vi "Current File Paths.vi"(5 "Analysis Mode":T1, 6 "Local Data in":T3, 7 "UI Refs":T2, 8 "error in (no error)":errorcluster) -> (0 "error out":errorcluster, 2 "Distances":dbl[](array[numeric]), 3 "Tags":string[](array[string]))   [LabVIEW 2024]
uses:
  Controls/RVHR - Local Data.ctl
  Controls/Test Cluster.ctl
  Controls/Excluded Information.ctl
  Controls/Language.ctl
  Controls/Device_Type.ctl
  <vilib>/Utility/miscctls.llb/LVRectTypeDef.ctl
  <vilib>/Utility/miscctls.llb/LVBoundsTypeDef.ctl
  Controls/RVHR - UI Refs.ctl
  Controls/RVHR - Analysis Mode.ctl
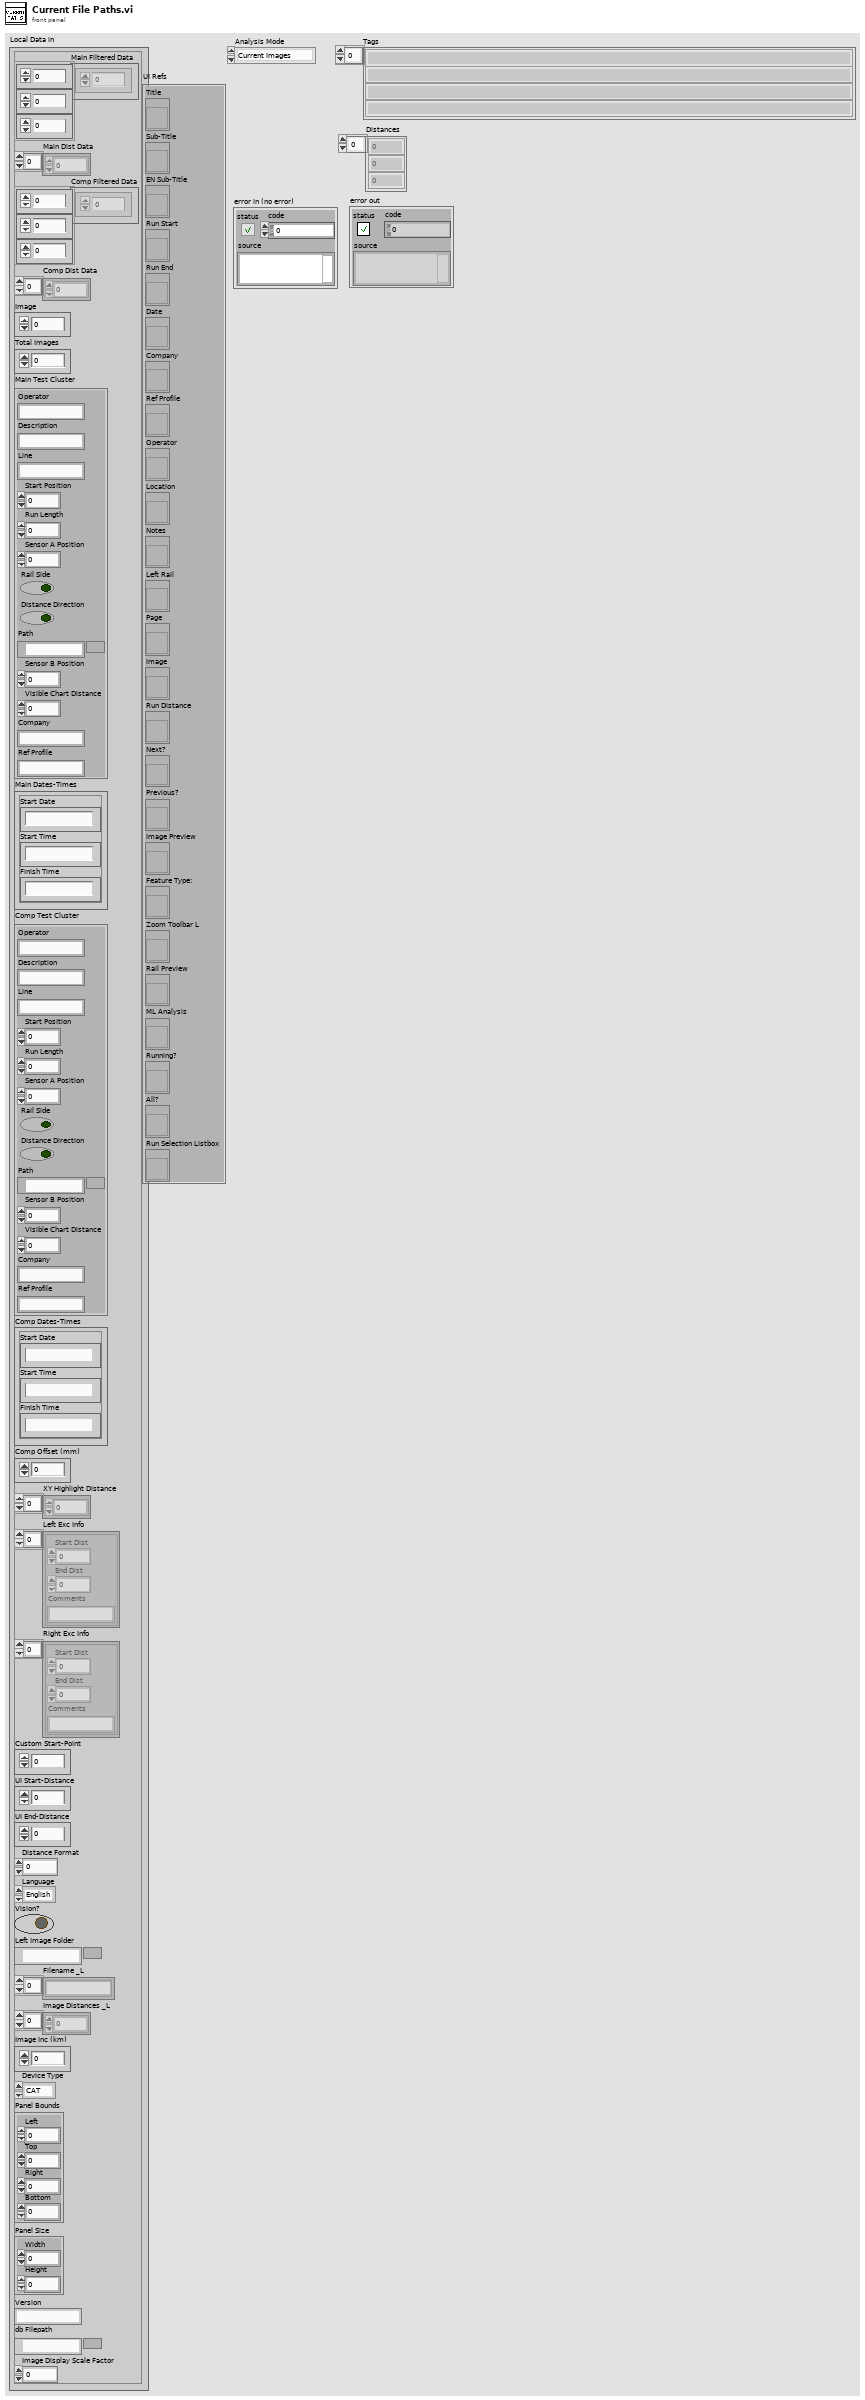
[diagram p1: front panel]
types:
  T1 = typedef "RVHR - Analysis Mode.ctl" = enum16{"Current Images", "Full Run"}
  T2 = typedef "RVHR - UI Refs.ctl" = cluster{"Title":refnum<vi>, "Sub-Title":refnum<vi>, "EN Sub-Title":refnum<vi>, "Run Start":refnum<vi>, "Run End":refnum<vi>, "Date":refnum<vi>, "Company":refnum<vi>, "Ref Profile":refnum<vi>, "Operator":refnum<vi>, "Location":refnum<vi>, "Notes":refnum<vi>, "Left Rail":refnum<vi>, "Page":refnum<vi>, "Image":refnum<vi>, "Run Distance":refnum<vi>, "Next?":refnum<vi>, "Previous?":refnum<vi>, "Image Preview":refnum<vi>, "Feature Type:":refnum<vi>, "Zoom Toolbar L":refnum<vi>, "Rail Preview":refnum<vi>, "ML Analysis":refnum<vi>, "Running?":refnum<vi>, "All?":refnum<vi>, "Run Selection Listbox":refnum<vi>}
  T3 = typedef "RVHR - Local Data.ctl" = cluster{"Main Filtered Data":dbl[][][], "Main Dist Data":dbl[], "Comp Filtered Data":dbl[][][], "Comp Dist Data":dbl[], "Image":u16, "Total Images":u16, "Main Test Cluster":T4, "Main Dates-Times":cluster{"Start Date":string, "Start Time":string, "Finish Time":string}, "Comp Test Cluster":T4, "Comp Dates-Times":cluster{"Start Date":string, "Start Time":string, "Finish Time":string}, "Comp Offset (mm)":i64, "XY Highlight Distance":dbl[], "Left Exc Info":T5[], "Right Exc Info":T5[], "Custom Start-Point":dbl, "UI Start-Distance":dbl, "UI End-Distance":dbl, "Distance Format":u8, "Language":T6, "Vision?":bool, "Left Image Folder":path, "Filename _L":string[], "Image Distances _L":dbl[], "Image Inc (km)":dbl, "Device Type":T7, "Panel Bounds":T8, "Panel Size":T9, "Version":string, "db Filepath":path, "Image Display Scale Factor":dbl}
  T4 = typedef "Test Cluster.ctl" = cluster{"Operator":string, "Description":string, "Line":string, "Start Position":dbl, "Run Length":dbl, "Sensor A Position":dbl, "Rail Side":bool, "Distance Direction":bool, "Path":path, "Sensor B Position":dbl, "Visible Chart Distance":dbl, "Company":string, "Ref Profile":string}
  T5 = typedef "Excluded Information.ctl" = cluster{"Start Dist":dbl, "End Dist":dbl, "Comments":string}
  T6 = typedef "Language.ctl" = enum16{"English", "Chinese", "German"}
  T7 = typedef "Device_Type.ctl" = enum16{"CAT", "Bi-CAT", "YRCA", "RCA", "RV-HR", "TV-HR"}
  T8 = typedef "LVRectTypeDef.ctl" = cluster{"Left":i16, "Top":i16, "Right":i16, "Bottom":i16}
  T9 = typedef "LVBoundsTypeDef.ctl" = cluster{"Width":u32, "Height":u32}
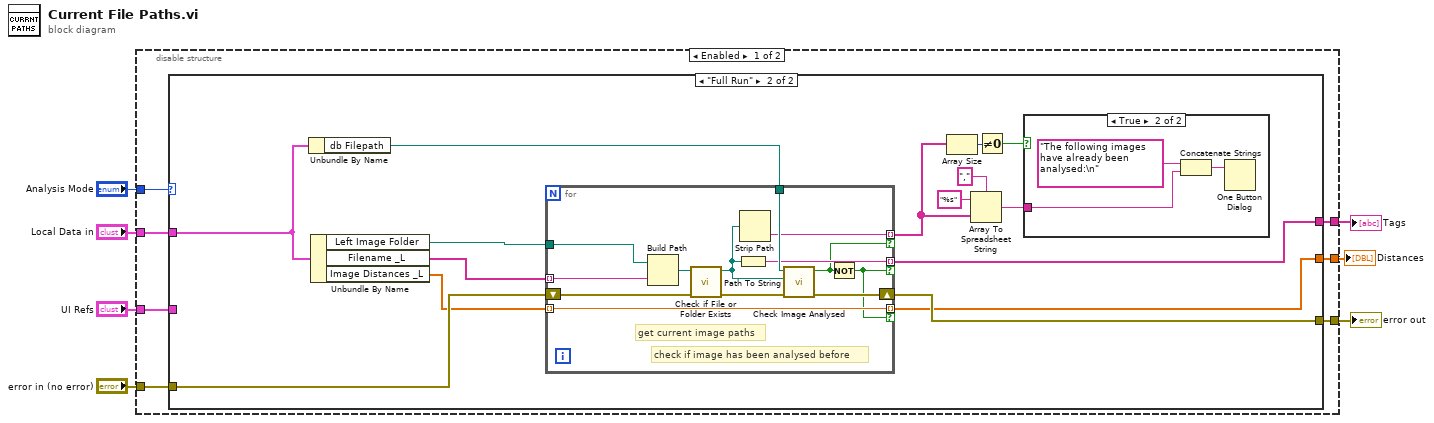
[diagram p0: block diagram]
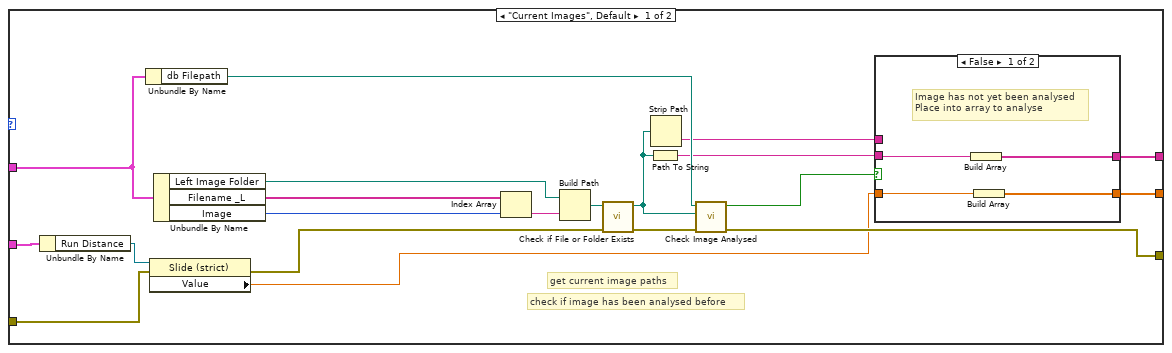
[diagram p2: hidden frame]
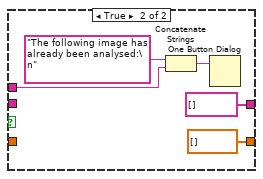
[diagram p3: hidden frame]
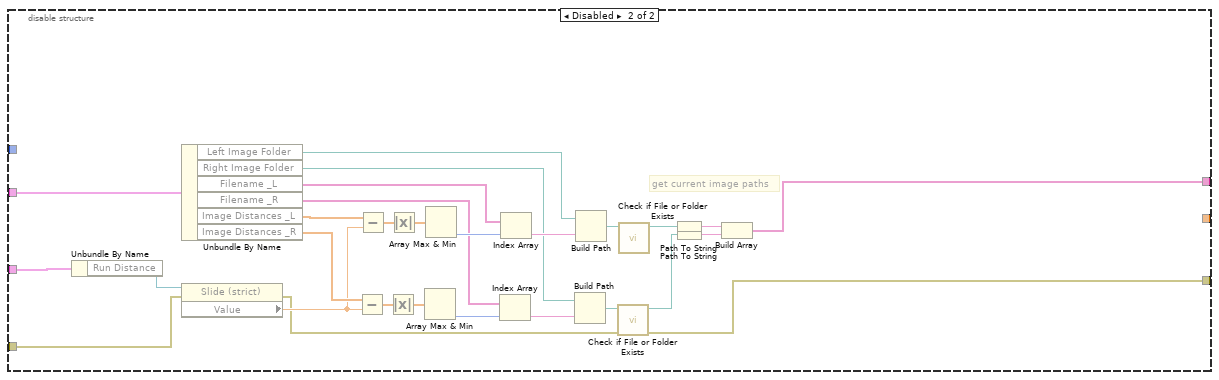
[diagram p5: hidden frame]
diagram:
  n1 = disable-structure shown="Enabled" {
    disable-tunnel: "Local Data in" -> [w10 w100]
    disable-tunnel: "UI Refs" -> [w14 w93]
    disable-tunnel: [w11 w78] -> w5
    disable-tunnel: [w12 w76] -> w4
    disable-tunnel: "error in (no error)" -> [w13 w75]
    disable-tunnel: "Analysis Mode" -> [w9 _]
    disable-tunnel: [w8 _] -> w1
    frame Enabled {
      n2 = case shown="\"Full Run\"" w9 {
        tunnel: w14 -> [w34 _]
        tunnel: w13 -> [w32 w58]
        tunnel: [w27 w55] -> w12
        tunnel: [w17 w54] -> w11
        tunnel: w10 -> [w26 w53]
        tunnel: [w15 w45] -> w8
        frame "Current Images", Default {
          # "get current image paths"
          # "check if image has been analysed before"
          n3 = Unbundle By Name(w34) -> ("Run Distance"=w33:refnum<vi>)
          n4 = Unbundle By Name(w26) -> ("db Filepath"=w25:path)
          n5 = property class="Slide (strict)"(reference=w33, error in=w32) -> (error out=w28:errorcluster, "Value"=w16:dbl)  [unwired: 1 out]
          n6 = Unbundle By Name(w26) -> ("Left Image Folder"=w31:path, "Filename _L"=w30:string[], "Image"=w29:u16)
          n7 = Index Array(array=w30, index=w29) -> (element=w23:string)
          n8 = Build Path(base path=w31, name or relative path=w23) -> (appended path=w22:path)
          n9 = call <vilib>:"Check if File or Folder Exists.vi"("error in (no error)"=w28, "path"=w22) -> ("error out"=w21:errorcluster, "dup path"=w20:path)  [unwired: 7 in, 1 out]
          n10 = Path To String(path=w20) -> (string=w18:string)
          n11 = Strip Path(path=w20) -> (name=w19:string)  [unwired: 1 out]
          n12 = call "Check Image Analysed.vi"("error in (no error)"=w21, "Image Path"=w20, "DB Path"=w25) -> ("error out"=w27:errorcluster, "analysed?"=w24:bool)  [unwired: 7 in]
          n13 = case shown="False" w24 {
            tunnel: w19 -> [_ w41]
            tunnel: w18 -> [w38 _]
            tunnel: [w37 string[] []] -> w17
            tunnel: w16 -> [w36 _]
            tunnel: [w35 dbl[] []] -> w15
            frame False {
              # "Image has not yet been analysed\nPlace into array to analyse"
              n14 = Build Array(w38) -> (w37:string[])
              n15 = Build Array(w36) -> (w35:dbl[])
            }
            frame True {
              n16 = Concatenate Strings("The following image has already been analysed:\n" ("string"), w41) -> (w42:string)
              n17 = One Button Dialog(message=w42) -> ()  [unwired: 1 in, 1 out]
            }
          }
        }
        frame "Full Run" {
          n18 = Unbundle By Name(w53) -> ("db Filepath"=w47:path)
          n19 = Unbundle By Name(w53) -> ("Left Image Folder"=w57:path, "Filename _L"=w56:string[], "Image Distances _L"=w46:dbl[])
          n20 = for {
            tunnel: w57 -> [w70]
            tunnel: w47 -> [w66]
            tunnel: [w65] -> w54 mode=indexing if=w59
            tunnel: [w63] -> w49 mode=indexing if=w61
            tunnel: w56 -> [w62] mode=indexing
            shift-right: [w68] -> w55
            shift-left: w58 -> [w67]
            tunnel: w46 -> [w60] mode=indexing
            tunnel: [w60] -> w45 mode=indexing if=w59
            # "get current image paths"
            # "check if image has been analysed before"
            n21 = Build Path(base path=w70, name or relative path=w62) -> (appended path=w71:path)
            n22 = call <vilib>:"Check if File or Folder Exists.vi"("error in (no error)"=w67, "path"=w71) -> ("error out"=w69:errorcluster, "dup path"=w64:path)  [unwired: 7 in, 1 out]
            n23 = Path To String(path=w64) -> (string=w65:string)
            n24 = Strip Path(path=w64) -> (name=w63:string)  [unwired: 1 out]
            n25 = call "Check Image Analysed.vi"("error in (no error)"=w69, "Image Path"=w64, "DB Path"=w66) -> ("error out"=w68:errorcluster, "analysed?"=w61:bool)  [unwired: 7 in]
            n26 = Not(x=w61) -> (.not. x?=w59:bool)
          }
          n27 = Array Size(array=w49) -> (size(s)=w52:i32)
          n28 = Array To Spreadsheet String(delimiter (Tab)=",", array=w49, 3:"%s" ("format string")) -> (spreadsheet string=w48:string)
          n29 = Not Equal To 0?(x=w52) -> (x != 0?=w44:bool)
          n30 = case shown="True" w44 {
            tunnel: w48 -> [_ w72]
            frame False {
            }
            frame True {
              n31 = Concatenate Strings("The following images have already been analysed:\n" ("string"), w72) -> (w73:string)
              n32 = One Button Dialog(message=w73) -> ()  [unwired: 1 in, 1 out]
            }
          }
        }
      }
    }
    frame Disabled {
      # "get current image paths"
      n33 = Unbundle By Name(w93) -> ("Run Distance"=w92:refnum<vi>)
      n34 = Unbundle By Name(w100) -> ("Left Image Folder"=w90:path, "Right Image Folder"=w81:path, "Filename _L"=w91:string[], "Filename _R"=w82:string[], "Image Distances _L"=w94:dbl[], "Image Distances _R"=w84:dbl[])
      n35 = property class="Slide (strict)"(reference=w92, error in=w75) -> (error out=w77:errorcluster, "Value"=w83:dbl)  [unwired: 1 out]
      n36 = Subtract(x=w84, y=w83) -> (x-y=w85:dbl[])
      n37 = Subtract(x=w94, y=w83) -> (x-y=w99:dbl[])
      n38 = Absolute Value(x=w85) -> (abs(x)=w86:dbl[])
      n39 = Absolute Value(x=w99) -> (abs(x)=w98:dbl[])
      n40 = Array Max & Min(array=w86) -> (min index (indices)=w87:i32)  [unwired: 3 out]
      n41 = Array Max & Min(array=w98) -> (min index (indices)=w97:i32)  [unwired: 3 out]
      n42 = Index Array(array=w82, index=w87) -> (element=w88:string)
      n43 = Index Array(array=w91, index=w97) -> (element=w96:string)
      n44 = Build Path(base path=w81, name or relative path=w88) -> (appended path=w89:path)
      n45 = Build Path(base path=w90, name or relative path=w96) -> (appended path=w95:path)
      n46 = call <vilib>:"Check if File or Folder Exists.vi"("error in (no error)"=w77, "path"=w89) -> ("error out"=w76:errorcluster, "dup path"=w79:path)  [unwired: 7 in, 1 out]
      n47 = call <vilib>:"Check if File or Folder Exists.vi"("path"=w95) -> ("dup path"=w80:path)  [unwired: 8 in, 2 out]
      n48 = Path To String(path=w80) -> (string=w102:string)
      n49 = Path To String(path=w79) -> (string=w101:string)
      n50 = Build Array(w102, w101) -> (w78:string[])
    }
  }
  "Tags" <- w5
  "error out" <- w4
  "Distances" <- w1
